vi "Controle_Dois_Motores_2.vi"() -> ()   [LabVIEW 2025]
panel:
  in  "Enable 3":tag
  in  "Direção 2":tag
  in  "Pulso 2":tag
  in  "Timer Reset":bool
  in  "stop":bool
  in  "Enable":bool
  in  "Direção  2":bool
  in  "Enable 2":tag
  in  "Direção":tag
  in  "Pulso":tag
  in  "Constante Calibracao (mm/pulsos)":dbl
  in  "Velocidade ( mm/s )":dbl
  in  "Distancia (mm)":dbl
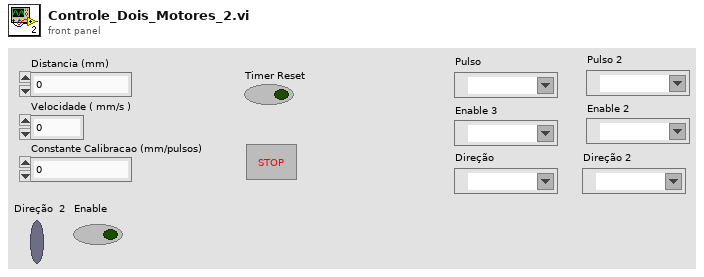
[diagram p1: front panel]
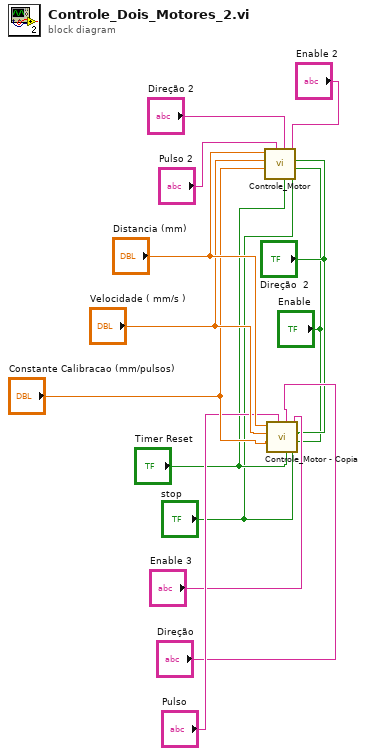
[diagram p0: block diagram]
diagram:
  n1 = call "Controle_Motor.vi"("stop"="stop", "Enable"="Enable", "Direção  2"="Direção  2", "Enable 2"="Enable 2", "Timer Reset"="Timer Reset", "Direção"="Direção 2", "Pulso"="Pulso 2", "Constante Calibracao (mm/pulsos)"="Constante Calibracao (mm/pulsos)", "Velocidade ( mm/s )"="Velocidade ( mm/s )", "Distancia (mm)"="Distancia (mm)") -> ()  [unwired: 2 in]
  n2 = call "Controle_Motor - Copia.vi"("stop"="stop", "Enable"="Enable", "Direção  2"="Direção  2", "Enable 2"="Enable 3", "Timer Reset"="Timer Reset", "Direção"="Direção", "Pulso"="Pulso", "Constante Calibracao (mm/pulsos)"="Constante Calibracao (mm/pulsos)", "Velocidade ( mm/s )"="Velocidade ( mm/s )", "Distancia (mm)"="Distancia (mm)") -> ()  [unwired: 2 in]
